vi "BLM control.vi"(2 "Point #":i32, 4 "Parameters":dbl[](array[numeric]) format="%.3e", 5 "Instrument Address":refnum<visa-resource-name>) -> (0 "Stop":bool, 1 "Data Out":dbl[](array[numeric]) format="%.2f")   [LabVIEW 2016]
doc: "Moves the stepper moter an appropriate amount based on the point number, step size and final position.\nScott Hannahs, NHMFL, March 1999"
uses:
  Serial Instruments/Serial Support VISA.llb/Serial Actions.ctl
panel:
  in  "Motor Address":string="0"
  in  "error in (no error)":errorcluster
  out "Starting Position":dbl format="%.2f"
  # "Motor Number"
  # "Step Size"
  # "Final Position"
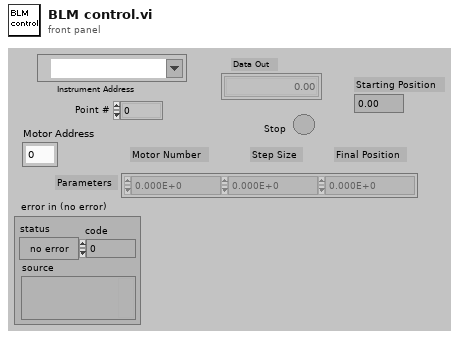
[diagram p1: front panel]
types:
  T1 = cluster{"Parameters[0]":dbl, "Parameters[1]":dbl, "Parameters[2]":dbl}
  T2 = typedef "Serial Actions.ctl" = enum16{"Init", "Break", "Clear Buffer", "Write", "Read", "N Bytes", "Lock", "Unlock", "Close"}
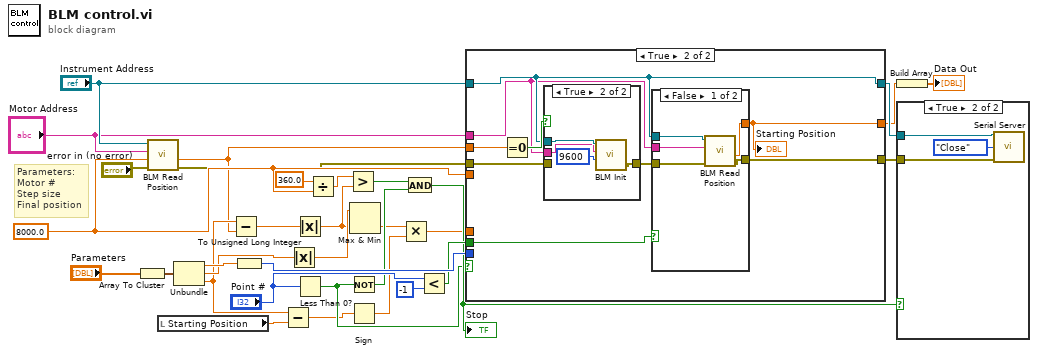
[diagram p0: block diagram]
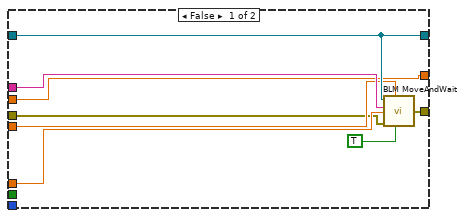
[diagram p3: hidden frame]
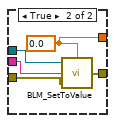
[diagram p5: hidden frame]
diagram:
  w13 = 8000.0 ("Steps/rot")
  # "Parameters:\nMotor #\nStep size\nFinal position"
  n1 = Array To Cluster(array="Parameters") -> (cluster=w32:T1)
  n2 = call "BLM Read Position.vi"("error in (no error)"="error in (no error)", "Steps/rot"=w13, "Motor Address"="Motor Address", "Port Address"="Instrument Address") -> ("error out"=w11:errorcluster, "Response"=w5:dbl)  [unwired: 2 out]
  n3 = local read "Starting Position"() -> (w9:dbl)
  n4 = Unbundle(w32) -> ("Parameters[0]"=w31:dbl, "Parameters[1]"=w24:dbl, "Parameters[2]"=w6:dbl)
  n5 = Subtract(x=w6, y=w5) -> (x-y=w4:dbl)
  n6 = To Unsigned Long Integer(number=w31) -> (unsigned 32bit integer=w28:u32)
  n7 = Subtract(x=w6, y=w9) -> (x-y=w8:dbl)
  n8 = Absolute Value(x=w24) -> (abs(x)=w3:dbl)
  n9 = Absolute Value(x=w4) -> (abs(x)=w2:dbl)
  n10 = Less Than 0?(x="Point #") -> (x < 0?=w20:bool)
  n11 = Divide(x=360.0, y=w13) -> (x/y=w1:dbl)
  n12 = Greater?(x=w1, y=w2) -> (0:w21:bool)
  n13 = Not(x=w20) -> (.not. x?=w19:bool)
  n14 = Sign(1:w8) -> (0:w23:dbl)
  n15 = Max & Min(x=w3, y=w2) -> (min(x,y)=w7:dbl)  [unwired: 1 out]
  n16 = Multiply(x=w7, y=w23) -> (x*y=w18:dbl)
  n17 = And(x=w21, y=w19) -> (x .and. y?=w22:bool)
  "Stop" <- w22
  n18 = Less?(x="Point #", y=-1) -> (x < y?=w25:bool)
  n19 = case shown="True" w20 {
    tunnel: "Instrument Address" -> [w38 w46]
    tunnel: [w38 w46] -> w29
    tunnel: w28 -> [_ _]
    tunnel: [w41 w50] -> w16
    tunnel: w25 -> [_ w49]
    tunnel: w18 -> [w40 _]
    tunnel: w13 -> [w36 _]
    tunnel: "Motor Address" -> [w37 w45]
    tunnel: [w35 w44] -> w17
    tunnel: w5 -> [w35 w43]
    tunnel: w11 -> [w34 w42]
    frame False {
      n20 = call "BLM MoveAndWait.vi"("Mode IS:"=TRUE ("Mode"), "Steps/rot"=w36, "error in (no error)"=w34, "Position / Distance"=w40, "Motor Address"=w37, "Instrument Address"=w38) -> ("error out"=w41:errorcluster)
    }
    frame True {
      n21 = Equal To 0?(x=w43) -> (x = 0?=w47:bool)
      n22 = case shown="True" w47 {
        tunnel: w46 -> [_ w54]
        tunnel: [w51 w53] -> w48
        tunnel: w45 -> [_ w52]
        tunnel: w42 -> [w51 _]
        frame False {
        }
        frame True {
          n23 = call "BLM Init.vi"("Baud Rate"=u32 9600, "Motor Address"=w52, "Port Address"=w54) -> ("error out"=w53:errorcluster)  [unwired: 1 in, 2 out]
        }
      }
      n24 = case shown="False" w49 {
        tunnel: w46 -> [w60 w65]
        tunnel: [w59 w64] -> w50
        tunnel: [w58 w61] -> w44
        tunnel: w48 -> [w57 w63]
        tunnel: w45 -> [w56 w62]
        frame False {
          n25 = call "BLM Read Position.vi"("error in (no error)"=w57, "Motor Address"=w56, "Port Address"=w60) -> ("error out"=w59:errorcluster, "Response"=w58:dbl)  [unwired: 1 in, 2 out]
        }
        frame True {
          w61 = 0.0
          n26 = call "BLM_SetToValue.vi"("Position"=w61, "error in (no error)"=w63, "Motor Address"=w62, "Port Address"=w65) -> ("error out"=w64:errorcluster)
        }
      }
      "Starting Position" <- w44
    }
  }
  n27 = Build Array(w17) -> (→"Data Out":dbl[])
  n28 = case shown="True" w22 {
    tunnel: w29 -> [_ w67]
    tunnel: w16 -> [_ w66]
    frame False {
    }
    frame True {
      n29 = call "Serial Server.vi"("VISA Resource Name"=w67, "Action"=Serial_Actions."Close", "error in (no error)"=w66) -> ()  [unwired: 8 in, 5 out]
    }
  }
